vi "Get Sorted Object Dictionary.vi"(11 "EDS in":refnum<class "EDS.lvclass">) -> (2 "Sorted Object Dictionary":refnum<class "Sorted Object Dictionary.lvclass">, 3 "EDS out":refnum<class "EDS.lvclass">)   [LabVIEW 2024, in "EDS.lvlib" / "EDS.lvclass"]
uses:
  EDS.lvclass
  Sorted Object Dictionary/Sorted Object Dictionary.lvclass
  EDS.lvclass/EDS.ctl
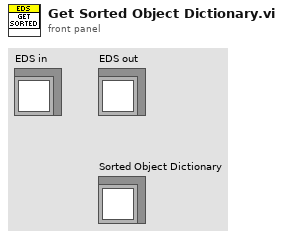
[diagram p1: front panel]
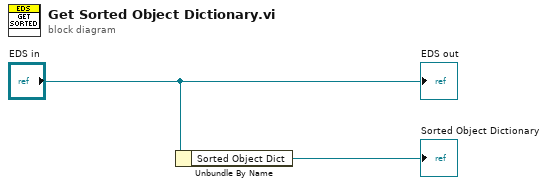
[diagram p0: block diagram]
diagram:
  n1 = Unbundle By Name("EDS in") -> ("Sorted Object Dict"=→"Sorted Object Dictionary":refnum<class "Sorted Object Dictionary.lvclass">)
  "EDS out" <- "EDS in"
